vi "Clear Data Sent Flag.vi"(5 "Component ID":u8, 7 "FPGA Interface":refnum<class "FPGA Interface.lvclass">, 8 "error in (no error)":errorcluster, 10 "Tx SubAddress (1-30)":u16, 11 "Remote Terminal in":refnum<class "Remote Terminal.lvclass">) -> (0 "error out":errorcluster)   [LabVIEW 2020, in "BCI-1553 API.lvlib" / "Remote Terminal.lvclass"]
doc: "Clears the current data sent flag from IC memory directly. The 'Data Sent' method will return false after this method is called, until a bus controller tells this remote terminal to transmit new data at the specified receive subaddress."
uses:
  Remote Terminal.lvclass
  Dependencies/FPGA Interface/FPGA Interface.lvclass
  Remote Terminal.lvclass/Remote Terminal.ctl
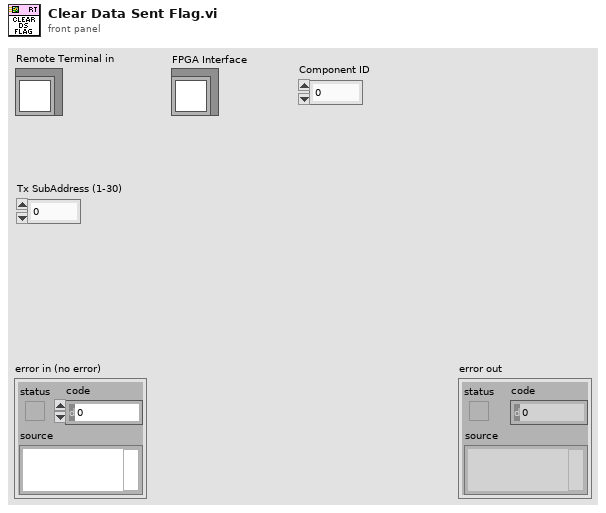
[diagram p1: front panel]
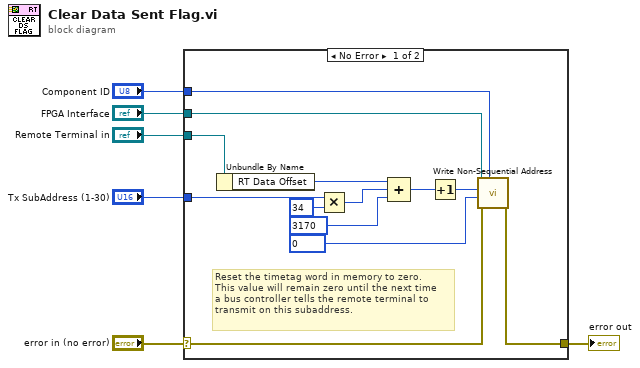
[diagram p0: block diagram]
diagram:
  n1 = case shown="No Error" "error in (no error)" {
    selector: "error in (no error)" -> [w8 w20]
    tunnel: [w7 w20] -> w5
    tunnel: "Remote Terminal in" -> [w12 _]
    tunnel: "FPGA Interface" -> [w19 _]
    tunnel: "Component ID" -> [w18 _]
    tunnel: "Tx SubAddress (1-30)" -> [w11 _]
    frame No Error {
      # "Reset the timetag word in memory to zero.\nThis value will remain zero until the next time\na bus controller tells the remote terminal to\ntransmit on this subaddress."
      n2 = Unbundle By Name(w12) -> ("RT Data Offset"=w16:u16)
      n3 = Multiply(x=w11, y=u16 34 ("Address")) -> (x*y=w15:u16)
      n4 = Compound Arithmetic op=ADD(w16, w15, u16 3170 ("Address")) -> (w17:u16)
      n5 = Increment(x=w17) -> (x+1=w10:u16)
      n6 = call-dynamic "Write Non-Sequential Address.vi"("Target IC (1-8)"=w18, "error in (no error)"=w8, "Data"=u16 0 ("Address"), "Address"=w10, "FPGA Interface in"=w19) -> ("error out"=w7:errorcluster)  [unwired: 6 in]
    }
    frame Error {
    }
  }
  "error out" <- w5
